vi "MissionGenerationTest.vi"() -> ()   [LabVIEW 2013]
doc: "A piece of test code to generate missions and add it to a queue without worrying about the network streams. Will not be used in the final.\n\n-3/5/2014 Elizabeth Mahon"
uses:
  Data/TypeDefs/UTM Location.ctl
  Data/TypeDefs/MissionTypeControl.ctl
  Classes/Missions/GoTo/GoTo.lvclass
  Classes/Missions/RoundBouy/RoundBouy.lvclass
  Classes/Missions/PassBouy/PassBouy.lvclass
  Classes/Missions/StationKeeping/StationKeeping.lvclass
  Classes/Missions/GenericMission/GenericMission.lvclass
panel:
  out "Points of Interest 2":T1[](array[typedef]) {"North" format="%#_10f"; "East" format="%#_8f"}
  out "Mission Type 2":T2
  in  "Pull from Q":bool
  in  "stop":bool
  in  "Mission Type":T2
  in  "Points of Interest":T1[](array[typedef]) {"North" format="%#_10f"; "East" format="%#_8f"}
  in  "Tolerance (m)":dbl
  in  "Duration (s)":dbl=-1.0
  in  "Timeout (s)":dbl=-1.0
  in  "OK Button":bool
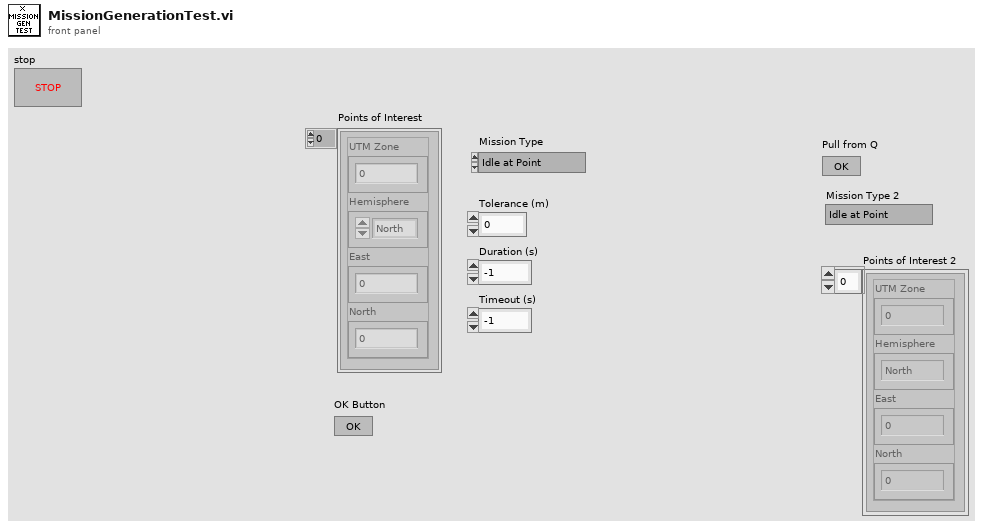
[diagram p1: front panel]
types:
  T1 = typedef "UTM Location.ctl" = cluster{"UTM Zone":dbl, "Hemisphere":enum16{"North", "South"}, "East":dbl, "North":dbl}
  T2 = typedef "MissionTypeControl.ctl" = enum16{"Idle at Point", "Drive to Waypoint", "Round Buoy to Port", "Round Buoy to Starboard", "Pass Between Buoys", "Station Keeping"}
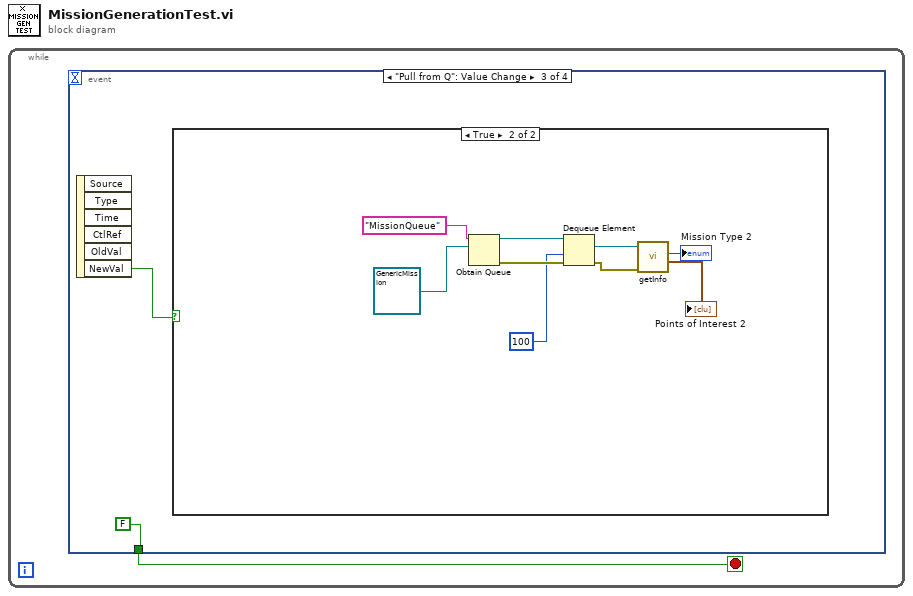
[diagram p0: block diagram]
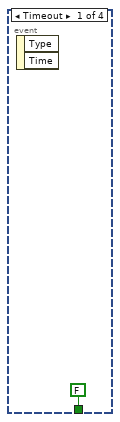
[diagram p2: hidden frame]
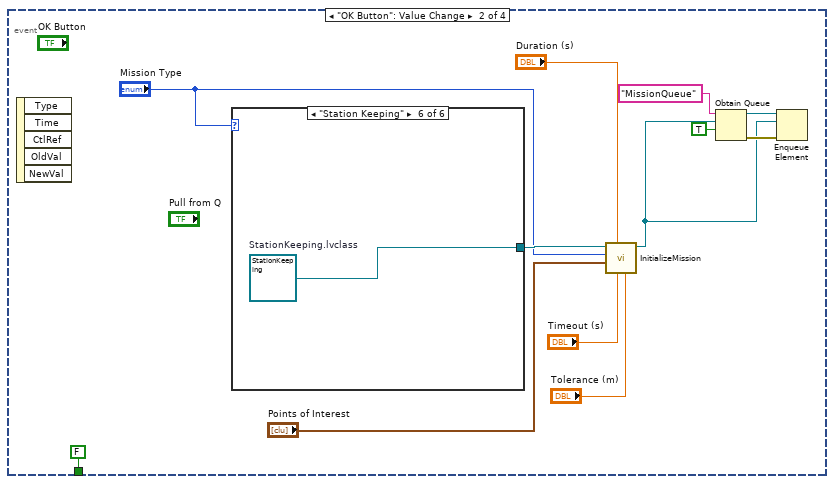
[diagram p3: hidden frame]
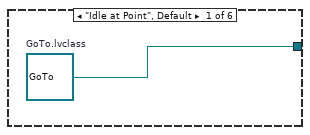
[diagram p4: hidden frame]
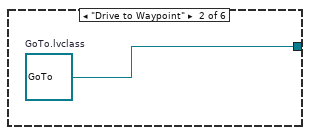
[diagram p5: hidden frame]
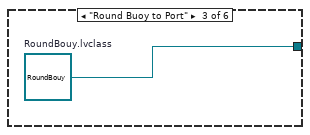
[diagram p6: hidden frame]
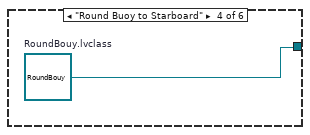
[diagram p7: hidden frame]
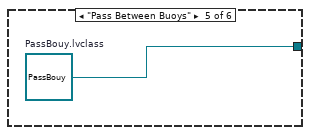
[diagram p8: hidden frame]
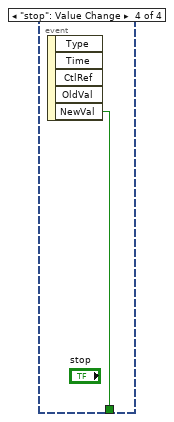
[diagram p10: hidden frame]
diagram:
  n1 = while {
    stop <- w1 stop-if-true
    n2 = event shown="[2] \"Pull from Q\": Value Change" {
      selector: _ -> [_ _ _ _]
      dyn-events: _ -> [_ _ _ _]
      timeout: _ -> [_ _ _ _]
      tunnel: [FALSE ("NewVal") FALSE ("NewVal") FALSE w32] -> w1
      event Timeout {
        n3 = event-data() -> ()  [unwired: 1 in, 2 out]
      }
      event "OK Button": Value Change {
        n4 = event-data() -> ()  [unwired: 1 in, 5 out]
        n5 = case shown="\"Station Keeping\"" "Mission Type" {
          tunnel: [w15 w16 w17 w18 w19 w20] -> w11
          frame "Idle at Point", Default {
            w15 = refnum<class "GoTo.lvclass"> refnum  # GoTo.lvclass
          }
          frame "Drive to Waypoint" {
            w16 = refnum<class "GoTo.lvclass"> refnum  # GoTo.lvclass
          }
          frame "Round Buoy to Port" {
            w17 = refnum<class "RoundBouy.lvclass"> refnum  # RoundBouy.lvclass
          }
          frame "Round Buoy to Starboard" {
            w18 = refnum<class "RoundBouy.lvclass"> refnum  # RoundBouy.lvclass
          }
          frame "Pass Between Buoys" {
            w19 = refnum<class "PassBouy.lvclass"> refnum  # PassBouy.lvclass
          }
          frame "Station Keeping" {
            w20 = refnum<class "StationKeeping.lvclass"> refnum  # StationKeeping.lvclass
          }
        }
        n6 = call-dynamic "InitializeMission.vi"("Tolerance (m)"="Tolerance (m)", "Timeout (s)"="Timeout (s)", "Duration (s)"="Duration (s)", "Points of Interest"="Points of Interest", "Mission Type"="Mission Type", "GenericMission in"=w11) -> ("GenericMission out"=w7:refnum<class "GenericMission.lvclass">)  [unwired: 4 in, 1 out]
        n7 = Obtain Queue(name (unnamed)="MissionQueue", element data type=w7, create if not found? (T)=TRUE) -> (queue out=w14:refnum<queue>, error out=w9:errorcluster)  [unwired: 2 in, 1 out]
        n8 = Enqueue Element(queue=w14, element=w7, error in (no error)=w9) -> ()  [unwired: 1 in, 3 out]
      }
      event "Pull from Q": Value Change {
        n9 = event-data() -> ("NewVal"=w22:bool)  [unwired: 1 in, 5 out]
        n10 = case shown="True" w22 {
          frame False {
          }
          frame True {
            n11 = Obtain Queue(name (unnamed)="MissionQueue", element data type=refnum<class "GenericMission.lvclass"> refnum ("GenericMission.lvclass")) -> (queue out=w29:refnum<queue>, error out=w30:errorcluster)  [unwired: 3 in, 1 out]
            n12 = Dequeue Element(queue=w29, timeout in ms (-1)=100, error in (no error)=w30) -> (element=w27:refnum<class "GenericMission.lvclass">, error out=w26:errorcluster)  [unwired: 2 out]
            n13 = call-dynamic "getInfo.vi"("error in (no error)"=w26, "GenericMission in"=w27) -> ("Points of Interest"=→"Points of Interest 2":T1[], "Mission Type"=→"Mission Type 2":T2)  [unwired: 2 in, 6 out]
          }
        }
      }
      event "stop": Value Change {
        n14 = event-data() -> ("NewVal"=w32:bool)  [unwired: 1 in, 4 out]
      }
    }
  }
